vi "normalize.vi"(11 "Array in":dbl[](array[numeric])) -> (3 "Array out":dbl[](array[numeric]))   [LabVIEW 2011]
uses:
  <vilib>/Analysis/NI_AALBase.lvlib
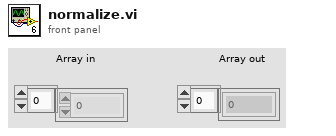
[diagram p1: front panel]
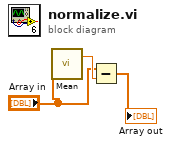
[diagram p0: block diagram]
diagram:
  n1 = call <vilib>:"Mean.vi"("X"="Array in") -> ("mean"=w2:dbl)  [unwired: 1 out]
  n2 = Subtract(x="Array in", y=w2) -> (x-y=→"Array out":dbl[])
